vi "RT_BLOGIC_InitDelay.vi"(9 "Dly_PT":u32, 10 "Err_In":errorcluster) -> (1 "Dly_Comp":bool, 2 "Err_Out":errorcluster)   [LabVIEW 2024]
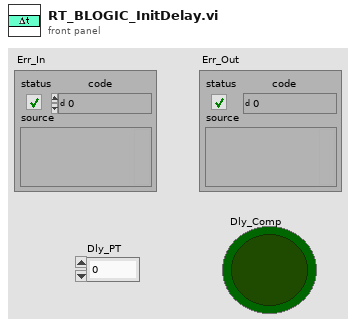
[diagram p1: front panel]
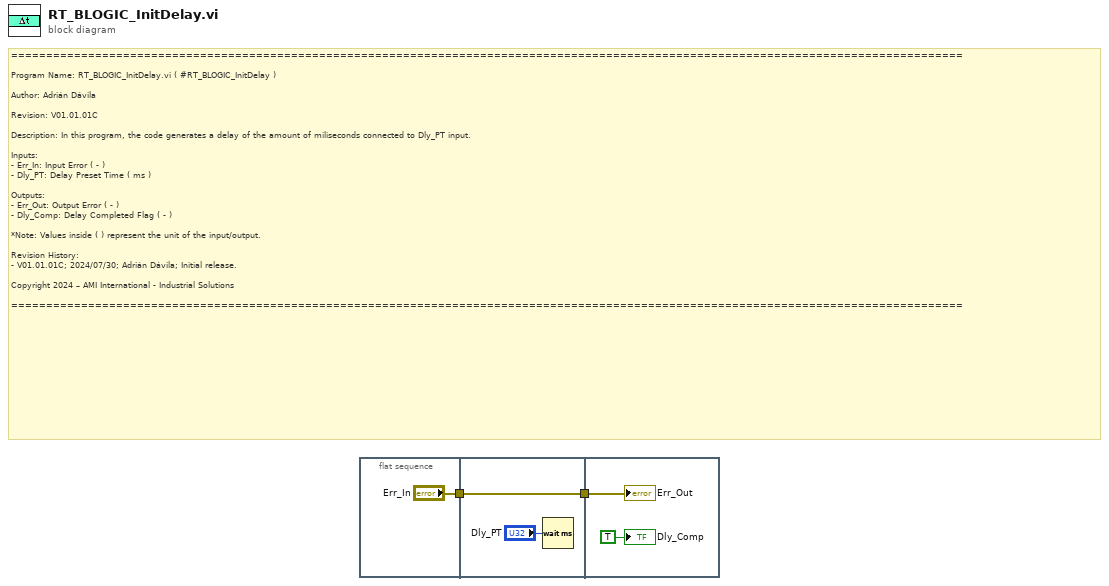
[diagram p0: block diagram]
diagram:
  # "========================================================================================================================================\n\nProgram Name: RT_BLOGIC_InitDelay.vi ( #RT_BLOGIC_InitDelay )\n\nAuthor: Adrián Dávila\n\nRevision: V01.01.01C\n\nDescription: In this program, the code generates a delay of the amount of miliseconds connected to Dly_PT input.\n\nInputs:\n- Err_In: Input Error ( - )\n- Dly_PT: Delay Preset Time ( ms )\n\nOutputs:\n- Err_Out: Output Error ( - )\n- Dly_Comp: Delay Completed Flag ( - )\n\n*Note: Values inside ( ) represent the unit of the input/output.\n \nRevision History: \n- V01.01.01C; 2024/07/30; Adrián Dávila; Initial release.  \n\nCopyright 2024 – AMI International - Industrial Solutions\n\n========================================================================================================================================"
  n1 = flat-sequence {
    tunnel: ["Err_In"] -> w1
    tunnel: [w4] -> w2
    tunnel: w1 -> [w4]
    tunnel: w2 -> [w7]
    frame #0 {
    }
    frame #1 {
      n2 = Wait (ms)(milliseconds to wait="Dly_PT") -> ()  [unwired: 1 out]
    }
    frame #2 {
      "Err_Out" <- w7
      "Dly_Comp" <- TRUE ("DONE")
    }
  }
